vi "Write Key.vi"(7 "section":string, 8 "error in (no error)":errorcluster, 9 "value":string, 10 "key":string) -> (0 "error out":errorcluster)   [LabVIEW 2020, in "Configuration Manager.lvclass"]
uses:
  Configuration Manager.lvclass
  <vilib>/Utility/config.llb/Write Key (String).vi
  Configuration Manager.lvclass/Configuration Manager.ctl
  <vilib>/Utility/config.llb/NI_LVConfig.lvlib
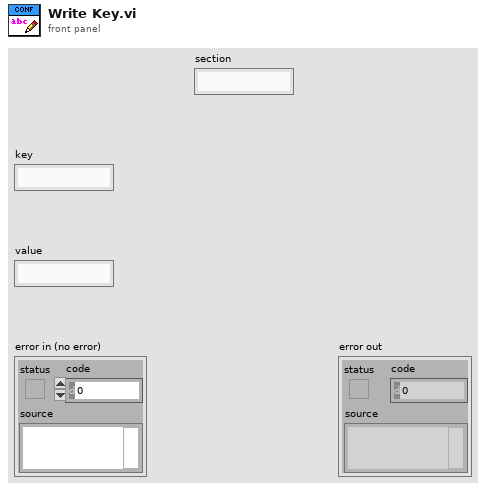
[diagram p1: front panel]
types:
  T1 = typedef "NI_LVConfig.lvlib/Config Data RefNum.ctl" = refnum<k1>
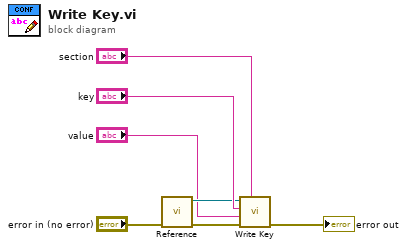
[diagram p0: block diagram]
diagram:
  n1 = call "Reference.vi"("error in (no error)"="error in (no error)") -> ("error out"=w6:errorcluster, "Refnum out"=w2:T1)  [unwired: 9 in]
  n2 = call-poly <vilib>:"Write Key.vi"("section"="section", "error in (no error)"=w6, "value"="value", "key"="key", "refnum"=w2) -> ("error out"=→"error out":errorcluster)  [unwired: 4 in, 2 out]
